vi "Update Map - View.vi"(8 "Column":i32, 9 "Row":i32, 10 "Updated View":i32[](array[numeric]) caption="Updated View (-1 team, 0 empty, 1 enemy)", 11 "map in":refnum<data-value>) -> (3 "map out":refnum<data-value>)   [LabVIEW 2017, in "DS Square.lvlib"]
uses:
  DS Square.lvlib
  Map.ctl
  Square Status.ctl
  Square State.ctl
  Center of Mass.ctl
  Common/Position.ctl
  SubVIs/Read-Only Globals.vi
  Square/Board Size.vi
  SubVIs/Globals (private).vi
  Common/Common.lvlib
  Square/Square.lvclass
panel:
  # "NW\nN\nNE\nE\nSE\nS\nSW\nW"
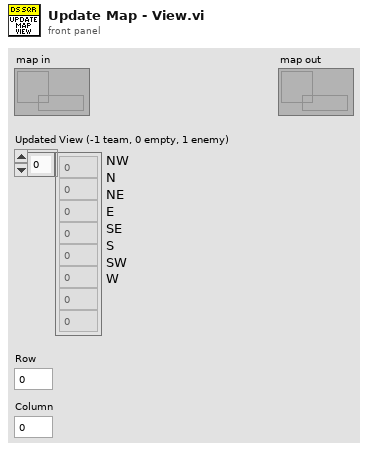
[diagram p1: front panel]
types:
  T1 = typedef "Common.lvlib/Position.ctl" = cluster{"Column":i32, "Row":i32}
  T2 = typedef "SB Type Defs.lvlib/Direction Enum.ctl" = enum16{"NW", "N", "NE", "E", "SE", "S", "SW", "W"}
  T3 = typedef "DS Square.lvlib/Square State.ctl" = enum16{"Unknown", "Empty", "Occupied - Active", "Occupied - Cool Down", "Attacked", "Enemy", "Enemy Wall"}
  T4 = typedef "DS Square.lvlib/Map.ctl" = cluster{"squares":T5[][], "center of mass":T6}
  T5 = typedef "DS Square.lvlib/Square Status.ctl" = cluster{"square state":T3, "probability":dbl, "last update":i32}
  T6 = typedef "DS Square.lvlib/Center of Mass.ctl" = cluster{"row":dbl, "col":dbl, "mass":dbl}
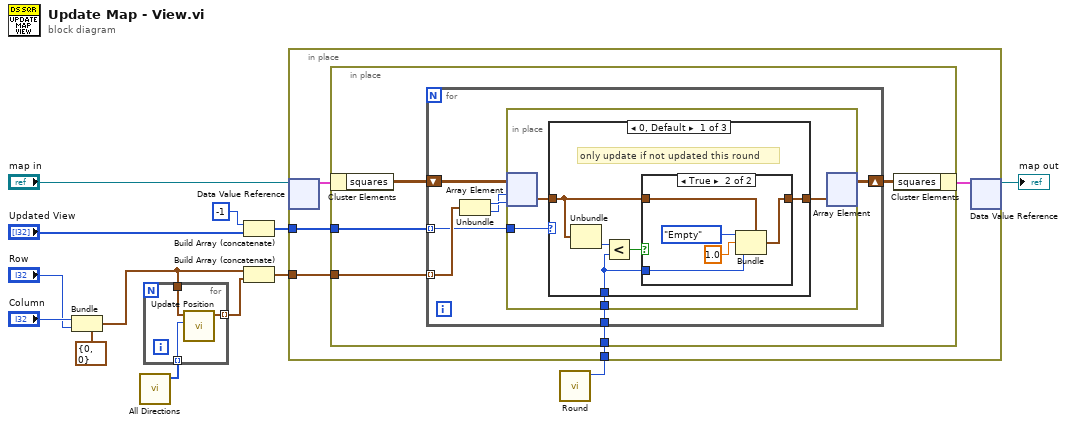
[diagram p0: block diagram]
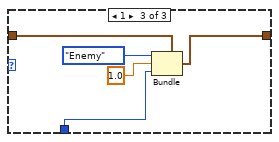
[diagram p4: hidden frame]
diagram:
  n1 = Bundle(cluster=T1 {"Column"=0, "Row"=0} ("Position in"), "Column"="Column", "Row"="Row") -> (w1:T1)
  n2 = call "All Directions.vi"() -> ("All directions"=w11:T2[])  [unwired: 11 in]
  n3 = for {
    tunnel: w1 -> [w16]
    tunnel: [w15] -> w9 mode=indexing
    tunnel: w11 -> [w14] mode=indexing
    n4 = call "Update Position.vi"("Direction"=w14, "Position in"=w16) -> ("Position out"=w15:T1)  [unwired: 9 in]
  }
  n5 = Build Array (concatenate)(-1 ("Numeric"), "Updated View") -> (w7:i32[])
  n6 = Build Array (concatenate)(w1, w9) -> (w8:T1[])
  n7 = call "Round.vi"() -> ("Round"=w10:i32)  [unwired: 11 in]
  n8 = in-place {
    in-place-border: w7 -> [w21]
    in-place-border: w8 -> [w20]
    in-place-border: w10 -> [w19]
    n9 = in-place-dvr #1("map in") -> (w18:T4)  [unwired: 1 out]
    n10 = in-place {
      in-place-border: w21 -> [w26]
      in-place-border: w20 -> [w25]
      in-place-border: w19 -> [w24]
      n11 = in-place-cluster #2(w18) -> ("squares"=w23:T5[][])
      n12 = for {
        tunnel: w26 -> [w29] mode=indexing
        shift-right: [w27] -> w22
        shift-left: w23 -> [w33]
        tunnel: w25 -> [w32] mode=indexing
        tunnel: w24 -> [w28]
        n13 = Unbundle(w32) -> ("Column"=w31:i32, "Row"=w30:i32)
        n14 = in-place {
          in-place-border: w29 -> [w37]
          in-place-border: w28 -> [w35]
          n15 = in-place-array #3(w33, w30, w31) -> (w36:T5)
          n16 = case shown="0, Default" w37 {
            tunnel: w36 -> [w41 w49 w54]
            tunnel: w35 -> [w40 _ w51]
            tunnel: [w42 w49 w50] -> w34
            frame 0, Default {
              # "only update if not updated this round"
              n17 = Unbundle(w41) -> ("last update"=w39:i32)  [unwired: 2 out]
              n18 = Less?(x=w39, y=w40) -> (x < y?=w38:bool)
              n19 = case shown="True" w38 {
                tunnel: [w43 w46] -> w42
                tunnel: w41 -> [w43 w45]
                tunnel: w40 -> [_ w44]
                frame False {
                }
                frame True {
                  n20 = Bundle(cluster=w45, "square state"=Square_State."Empty", "probability"=1.0, "last update"=w44) -> (w46:T5)
                }
              }
            }
            frame -1 {
              # "don't update this...\nlast update indicates\nhow much longer cool\ndown will last"
            }
            frame 1 {
              n21 = Bundle(cluster=w54, "square state"=Square_State."Enemy", "probability"=1.0, "last update"=w51) -> (w50:T5)
            }
          }
          n22 = in-place-array #3(w34) -> (w27:T5[][])  [unwired: 2 out]
        }
      }
      n23 = in-place-cluster #2("squares"=w22) -> (w17:T4)
    }
    n24 = in-place-dvr #1(w17) -> (→"map out":refnum<data-value>)  [unwired: 1 out]
  }
